vi "Set Active Channel.vi"(8 "error in":errorcluster, 10 "Channel":T1, 11 "2936r in":refnum<class "2936r.lvclass">) -> (0 "error out":errorcluster, 3 "2936r out":refnum<class "2936r.lvclass">)   [LabVIEW 2018, in "2936r.lvlib" / "2936r.lvclass"]
uses:
  2936r.lvclass
  PPLs/Optical Power Meter/Optical Power Meter.lvlibp/Custom Controls/Channel List.ctl
  2936r.lvclass/2936r.ctl
  PPLs/Optical Power Meter/Optical Power Meter.lvlibp
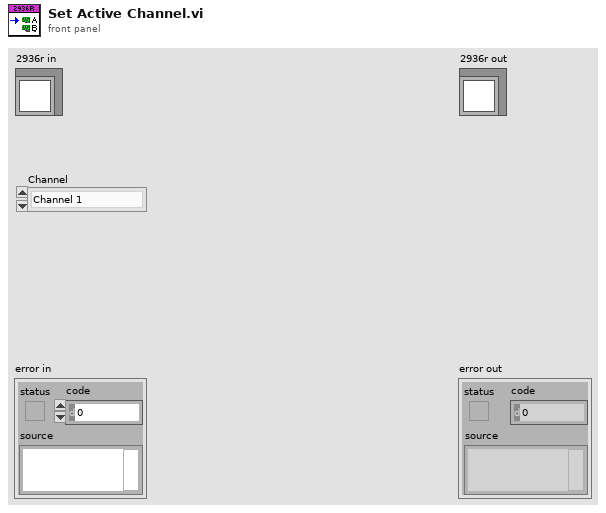
[diagram p1: front panel]
types:
  T1 = typedef "Optical Power Meter.lvlibp/Channel List.ctl" = enum16{"Channel 1", "Channel 2", "Channel 3", "Channel 4"}
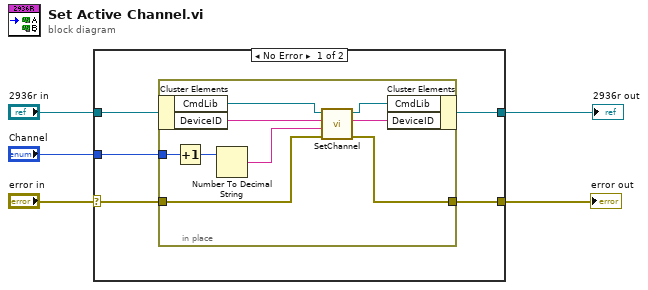
[diagram p0: block diagram]
diagram:
  n1 = case shown="No Error" "error in" {
    selector: "error in" -> [w8 w21]
    tunnel: [w10 w21] -> w4
    tunnel: [w6 w20] -> w2
    tunnel: "2936r in" -> [w7 w20]
    tunnel: "Channel" -> [w9 _]
    frame No Error {
      n2 = in-place {
        in-place-border: [w19] -> w10
        in-place-border: w9 -> [w18]
        in-place-border: w8 -> [w16]
        n3 = in-place-cluster #1(w7) -> ("CmdLib"=w14:refnum<k24>, "DeviceID"=w13:string)
        n4 = Increment(x=w18) -> (x+1=w17:T1)
        n5 = Number To Decimal String(number=w17) -> (decimal integer string=w15:string)  [unwired: 1 in]
        n6 = call <instrlib>:"SetChannel.vi"("error in"=w16, "Channel 1 or 2"=w15, "Device Key In"=w13, "PM Cmds In"=w14) -> ("error out"=w19:errorcluster, "Device Key Out"=w11:string, "PM Cmds Out"=w12:refnum<k24>)  [unwired: 1 in]
        n7 = in-place-cluster #1("CmdLib"=w12, "DeviceID"=w11) -> (w6:refnum<class "2936r.lvclass">)
      }
    }
    frame Error {
    }
  }
  "error out" <- w4
  "2936r out" <- w2
